vi "ECAT Download Firmware Progress.vi"(4 "Device Filename":string, 5 "Slave Ref":refnum<k21>, 6 "ShowFront?":bool, 7 "NeedReset":bool=TRUE, 8 "error in":errorcluster, 9 "File Byte Array":u8[](array[numeric])) -> (0 "Error Out":errorcluster)   [LabVIEW 2020, in "SEECD System Explorer.lvlib"]
uses:
  SEECD System Explorer.lvlib
  <vilib>/Utility/error.llb/DialogType.ctl
panel:
  out "Downloading....":u8(slide) caption="Downloading..." scale=0.0..118.0
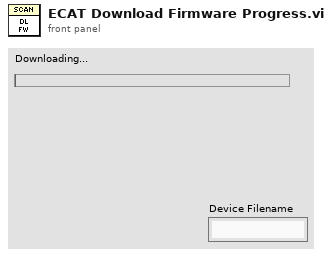
[diagram p1: front panel]
types:
  T1 = typedef "DialogType.ctl" = u16
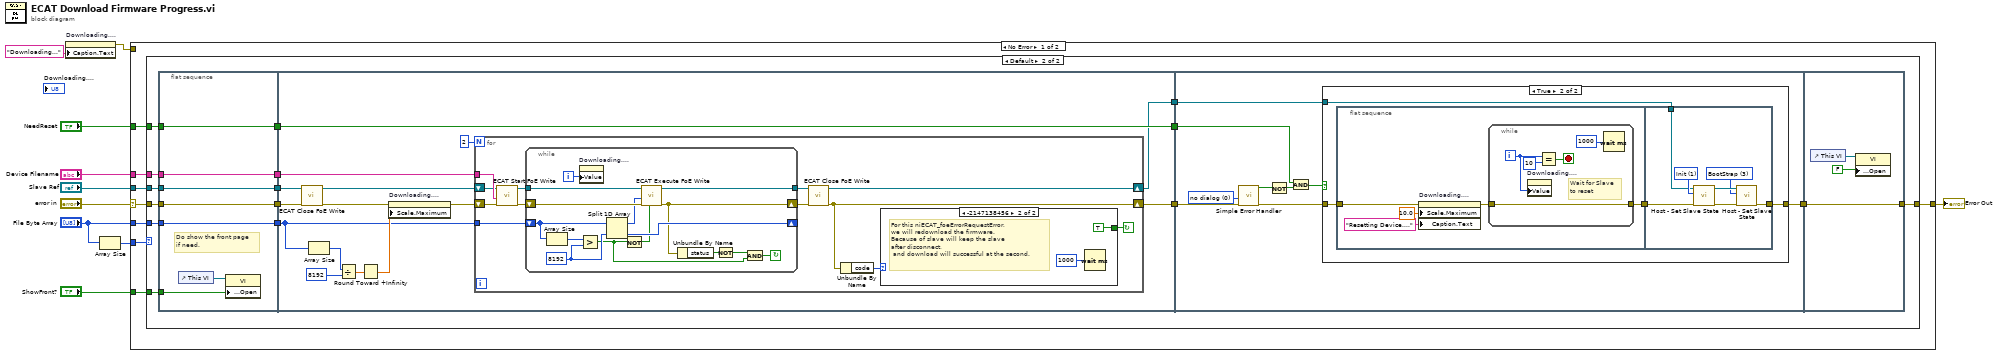
[diagram p0: block diagram]
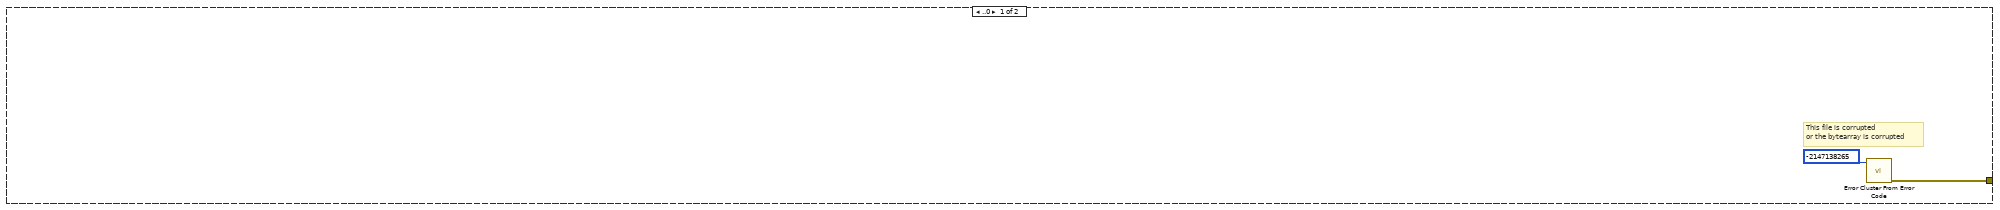
[diagram p2: hidden frame]
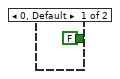
[diagram p3: hidden frame]
diagram:
  n1 = property on="Downloading...." class="Slide (strict)"("Caption.Text"="Downloading...") -> (error out=w8:errorcluster)  [unwired: 2 in, 1 out]
  n2 = Array Size(array="File Byte Array") -> (size(s)=w3:i32)
  n3 = case shown="No Error" "error in" {
    selector: "error in" -> [w13 w123]
    tunnel: [w17 w123] -> w10
    tunnel: w8 -> [_ _]
    tunnel: "ShowFront?" -> [w18 _]
    tunnel: "File Byte Array" -> [w16 _]
    tunnel: "NeedReset" -> [w15 _]
    tunnel: w3 -> [w14 _]
    tunnel: "Slave Ref" -> [w12 _]
    tunnel: "Device Filename" -> [w11 _]
    frame No Error {
      n4 = case shown="Default" w14 {
        tunnel: w18 -> [_ w30]
        tunnel: [w19 w29] -> w17
        tunnel: w16 -> [_ w28]
        tunnel: w15 -> [_ w27]
        tunnel: w13 -> [_ w26]
        tunnel: w12 -> [_ w25]
        tunnel: w11 -> [_ w22]
        frame ..0 {
          # "This file is corrupted\nor the bytearray is corrupted"
          n5 = call <vilib>:"Error Cluster From Error Code.vi"("error code (0)"=-2147138265) -> ("error out"=w19:errorcluster)  [unwired: 8 in]
        }
        frame Default {
          n6 = flat-sequence {
            tunnel: w26 -> [w43]
            tunnel: [w43] -> w36
            tunnel: w30 -> [w41]
            tunnel: [w40] -> w35
            tunnel: w28 -> [w40]
            tunnel: w27 -> [w39]
            tunnel: [w39] -> w34
            tunnel: w25 -> [w38]
            tunnel: [w38] -> w24
            tunnel: [w37] -> w23
            tunnel: w22 -> [w37]
            tunnel: [w58] -> w33
            tunnel: w36 -> [w55]
            tunnel: w35 -> [w49]
            tunnel: w34 -> [w48]
            tunnel: [w48] -> w32
            tunnel: w24 -> [w46]
            tunnel: w23 -> [w47]
            tunnel: [w44] -> w21
            tunnel: w33 -> [w95]
            tunnel: [w97] -> w31
            tunnel: w32 -> [w96]
            tunnel: w21 -> [w89]
            tunnel: [w122] -> w29
            tunnel: w31 -> [w122]
            frame #0 {
              # "Do show the front page\nif need."
              n7 = control-ref of="This VI"() -> (w42:refnum<vi>)
              n8 = property class="VI"(reference=w42, "Front Panel.Open"=w41) -> ()  [unwired: 1 in, 2 out]
            }
            frame #1 {
              n9 = call "ECAT Close FoE Write.vi"("Error In"=w55, "Slave Ref in"=w46) -> ("Error Out"=w54:errorcluster, "Slave Ref out"=w45:refnum<k21>)  [unwired: 3 in, 5 out]
              n10 = Array Size(array=w49) -> (size(s)=w53:i32)
              n11 = Divide(x=w53, y=8192) -> (x/y=w51:dbl)
              n12 = Round Toward +Infinity(x=w51) -> (ceil(x): smallest int >= x=w50:dbl)
              n13 = property on="Downloading...." class="Slide (strict)"(error in=w54, "Scale.Maximum"=w50) -> (error out=w56:errorcluster)  [unwired: 1 in, 1 out]
              n14 = for {
                N: 2 -> [_]
                tunnel: w47 -> [w66]
                tunnel: w49 -> [w65]
                shift-right: [w59] -> w44
                shift-left: w45 -> [w62]
                shift-right: [w64] -> w58
                shift-left: w56 -> [w68]
                stop <- w69 continue-if-true
                n15 = call "ECAT Start FoE Write.vi"("error in"=w68, "Device Filename"=w66, "Slave Ref in"=w62) -> ("error out"=w67:errorcluster, "Slave Ref out"=w61:refnum<k21>)  [unwired: 2 in, 5 out]
                n16 = while {
                  shift-right: [w80] -> w63
                  shift-left: w67 -> [w88]
                  shift-right: [w83] -> _
                  shift-left: w65 -> [w85]
                  tunnel: w61 -> [w75]
                  tunnel: [w74] -> w60
                  i -> [w87]
                  stop <- w76 continue-if-true
                  w84 = 8192 ("y")
                  n17 = Array Size(array=w85) -> (size(s)=w86:i32)
                  n18 = property on="Downloading...." class="Slide (strict)"("Value"=w87) -> ()  [unwired: 2 in, 2 out]
                  n19 = Greater?(x=w86, y=w84) -> (0:w77:bool)
                  n20 = Split 1D Array(array=w85, index=w84) -> (first subarray=w81:u8[], second subarray=w83:u8[])
                  n21 = Not(x=w77) -> (.not. x?=w82:bool)
                  n22 = call "ECAT Execute FoE Write.vi"("Finish"=w82, "error In"=w88, "File Byte Array"=w81, "Slave Ref in"=w75) -> ("error Out"=w80:errorcluster, "Slave Ref out"=w74:refnum<k21>)  [unwired: 3 in, 3 out]
                  n23 = Unbundle By Name(w80) -> ("status"=w79:bool)
                  n24 = Not(x=w79) -> (.not. x?=w78:bool)
                  n25 = And(x=w78, y=w77) -> (x .and. y?=w76:bool)
                }
                n26 = call "ECAT Close FoE Write.vi"("Error In"=w63, "Slave Ref in"=w60) -> ("Error Out"=w64:errorcluster, "Slave Ref out"=w59:refnum<k21>)  [unwired: 3 in, 5 out]
                n27 = Unbundle By Name(w64) -> ("code"=w70:i32)
                n28 = case shown="-2147138456" w70 {
                  tunnel: [FALSE TRUE] -> w69
                  frame 0, Default {
                  }
                  frame -2147138456 {
                    # "For this niECAT_foeErrorRequestError,\nwe will redownload the firmware.\nBecause of slave will keep the slave \nafter disconnect,\n and download will successful at the second."
                    n29 = Wait (ms)(milliseconds to wait=u32 1000) -> ()  [unwired: 1 out]
                  }
                }
              }
            }
            frame #2 {
              w90 = T1 0 items=["no dialog", "OK message", "continue or stop message", "OK message + warnings", "continue/stop + warnings"] ("type of dialog (OK msg:1)")
              n30 = call <vilib>:"Simple Error Handler.vi"("type of dialog (OK msg:1)"=w90, "error in (no error)"=w95) -> ("error?"=w92:bool, "error out"=w93:errorcluster)  [unwired: 3 in, 3 out]
              n31 = Not(x=w92) -> (.not. x?=w91:bool)
              n32 = And(x=w96, y=w91) -> (x .and. y?=w94:bool)
              n33 = case shown="True" w94 {
                tunnel: [w98 w102] -> w97
                tunnel: w93 -> [w98 w100]
                tunnel: w89 -> [_ w99]
                frame False {
                }
                frame True {
                  n34 = flat-sequence {
                    tunnel: [w106] -> w101
                    tunnel: w100 -> [w103]
                    tunnel: [w116] -> w102
                    tunnel: w101 -> [w115]
                    tunnel: w99 -> [w113]
                    frame #0 {
                      n35 = property on="Downloading...." class="Slide (strict)"(error in=w103, "Scale.Maximum"=10.0 ("Scale.Range:Maximum"), "Caption.Text"="Resetting Device....") -> (error out=w107:errorcluster)  [unwired: 1 in, 1 out]
                      n36 = while {
                        tunnel: w107 -> [w111]
                        tunnel: [w111] -> w106
                        i -> [w110]
                        stop <- w108 stop-if-true
                        # "Wait for Slave to reset"
                        n37 = property on="Downloading...." class="Slide (strict)"("Value"=w110) -> ()  [unwired: 2 in, 2 out]
                        n38 = Equal?(x=w110, y=10) -> (x = y?=w108:bool)
                        n39 = Wait (ms)(milliseconds to wait=u32 1000) -> ()  [unwired: 1 out]
                      }
                    }
                    frame #1 {
                      w117 = u32 3 items=["Init"=1, "PreOP"=2, "BootStrap"=3, "SafeOP"=4, "OP"=8] ("slaveState")
                      w119 = u32 1 items=["Init"=1, "PreOP"=2, "BootStrap"=3, "SafeOP"=4, "OP"=8] ("slaveState")
                      n40 = call "Host - Set Slave State.vi"("error in (no error)"=w115, "slaveState"=w119, "Slave Ref in"=w113) -> ("error out"=w114:errorcluster, "Slave Ref out"=w118:refnum<k21>)  [unwired: 5 in, 2 out]
                      n41 = call "Host - Set Slave State.vi"("error in (no error)"=w114, "slaveState"=w117, "Slave Ref in"=w118) -> ("error out"=w116:errorcluster)  [unwired: 5 in, 3 out]
                    }
                  }
                }
              }
            }
            frame #3 {
              n42 = control-ref of="This VI"() -> (w121:refnum<vi>)
              n43 = property class="VI"(reference=w121, "Front Panel.Open"=FALSE ("Front Panel Window:Open")) -> ()  [unwired: 1 in, 2 out]
            }
          }
        }
      }
    }
    frame Error {
    }
  }
  "Error Out" <- w10
